vi "ACR_STATUS.vi"(7 "EnableDrive":bool, 8 "error in (no error)":errorcluster, 9 "bstrRequest":string="p4360", 10 "nBit":i32=8465, 11 "Automation Refnum in":refnum<k7>) -> (0 "error out":errorcluster, 2 "DrvEnaOut":bool, 3 "Automation Refnum out":refnum<k7>)   [LabVIEW 2015]
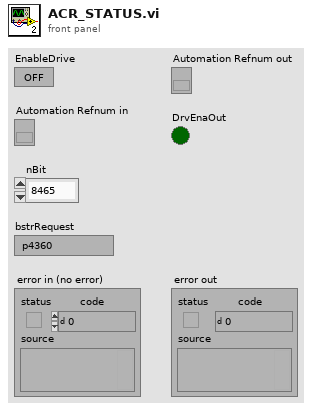
[diagram p1: front panel]
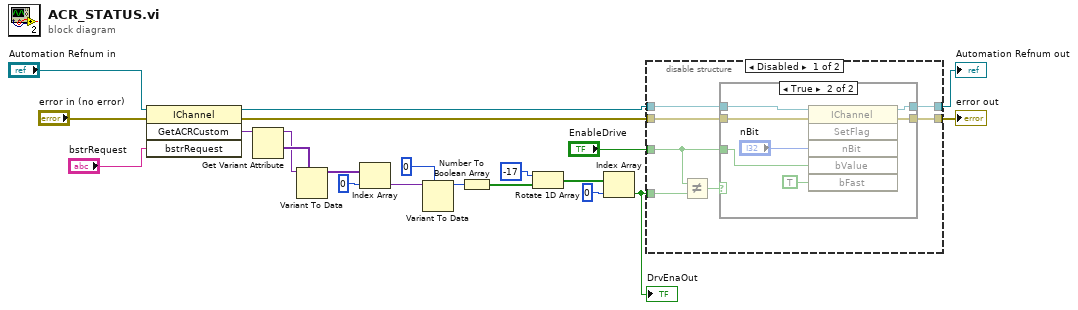
[diagram p0: block diagram]
diagram:
  n1 = invoke class="IChannel" method="GetACRCustom"(reference="Automation Refnum in", error in="error in (no error)", "bstrRequest"="bstrRequest") -> (reference out=w18:refnum<k7>, error out=w19:errorcluster, "GetACRCustom"=w9:variant)  [unwired: 1 in, 1 out]
  n2 = Get Variant Attribute(Variant=w9) -> (duplicate Variant=w5:variant, values=w6:variant[])  [unwired: 1 in, 4 out]
  n3 = Variant To Data(type=w6, Variant=w5) -> (data=w8:variant[])  [unwired: 1 in, 1 out]
  n4 = Index Array(array=w8, index=0 ("Index")) -> (element=w3:variant)
  n5 = Variant To Data(type=0, Variant=w3) -> (data=w16:i32)  [unwired: 1 in, 1 out]
  n6 = Number To Boolean Array(number=w16) -> (Boolean array=w12:bool[])
  n7 = Rotate 1D Array(1:w12, 2:-17 ("n")) -> (0:w17:bool[])
  n8 = Index Array(array=w17, index=0 ("Index")) -> (element=w15:bool)
  "DrvEnaOut" <- w15
  n9 = disable-structure shown="Disabled" {
    disable-tunnel: w15 -> [w28 _]
    disable-tunnel: w18 -> [w26 _]
    disable-tunnel: w19 -> [w25 _]
    disable-tunnel: [w24 _] -> w20
    disable-tunnel: [w23 _] -> w21
    disable-tunnel: "EnableDrive" -> [w22 _]
    frame Disabled {
      n10 = Not Equal?(x=w22, y=w28) -> (x != y?=w27:bool)
      n11 = case shown="True" w27 {
        tunnel: w22 -> [_ w36]
        tunnel: w26 -> [w30 w35]
        tunnel: w25 -> [w29 w34]
        tunnel: [w30 w33] -> w24
        tunnel: [w29 w32] -> w23
        frame False {
        }
        frame True {
          n12 = invoke class="IChannel" method="SetFlag"(reference=w35, error in=w34, "nBit"="nBit", "bValue"=w36, "bFast"=TRUE) -> (reference out=w33:refnum<k7>, error out=w32:errorcluster)  [unwired: 1 in, 4 out]
        }
      }
    }
    frame Enabled {
    }
  }
  "Automation Refnum out" <- w20
  "error out" <- w21
